vi "Tosca-Set Sequential Order.vi"(0 "Nx":i32, 5 "Ny":i32, 9 "N":i32) -> (4 "ix":i32[](array[numeric]), 6 "iy":i32[](array[numeric]))   [LabVIEW 2020]
uses:
  epl-vi-lib/Utility VIs/Math VIs/LinSpace (x0-dx-npts).vi
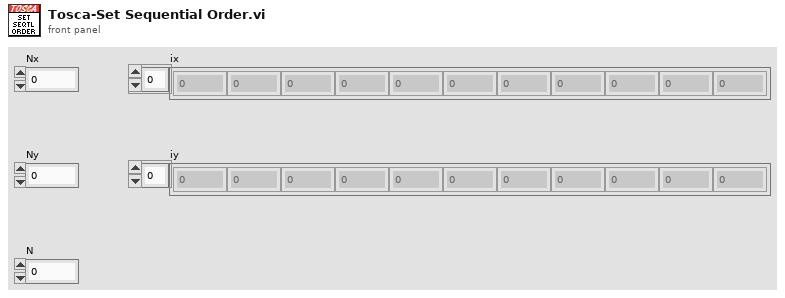
[diagram p1: front panel]
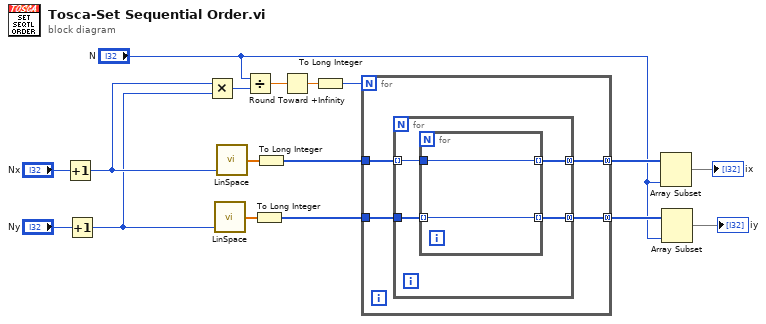
[diagram p0: block diagram]
diagram:
  n1 = Increment(x="Nx") -> (x+1=w3:i32)
  n2 = Increment(x="Ny") -> (x+1=w1:i32)
  n3 = Multiply(x=w3, y=w1) -> (x*y=w13:i32)
  n4 = call-poly "LinSpace.vi"("npts"=w1) -> ("Array"=w17:dbl[])  [unwired: 3 in, 1 out]
  n5 = call-poly "LinSpace.vi"("npts"=w3) -> ("Array"=w16:dbl[])  [unwired: 3 in, 1 out]
  n6 = Divide(x="N", y=w13) -> (x/y=w12:dbl)
  n7 = To Long Integer(number=w17) -> (32bit integer=w14:i32[])
  n8 = To Long Integer(number=w16) -> (32bit integer=w15:i32[])
  n9 = Round Toward +Infinity(x=w12) -> (ceil(x): smallest int >= x=w11:dbl)
  n10 = To Long Integer(number=w11) -> (32bit integer=w10:i32)
  n11 = for {
    N: w10 -> [_]
    tunnel: w15 -> [w21]
    tunnel: w14 -> [w20]
    tunnel: [w19] -> w9 mode=concatenating
    tunnel: [w18] -> w8 mode=concatenating
    n12 = for {
      tunnel: w21 -> [w24] mode=indexing
      tunnel: w20 -> [w25]
      tunnel: [w23] -> w19 mode=concatenating
      tunnel: [w22] -> w18 mode=concatenating
      n13 = for {
        tunnel: w25 -> [w26] mode=indexing
        tunnel: w24 -> [w27]
        tunnel: [w27] -> w23 mode=indexing
        tunnel: [w26] -> w22 mode=indexing
      }
    }
  }
  n14 = Array Subset(array=w9, length="N") -> (→"ix":i32[])  [unwired: 1 in]
  n15 = Array Subset(array=w8, length="N") -> (→"iy":i32[])  [unwired: 1 in]
